vi "LINC Command Lookup.vi"(8 "error in (no error)":errorcluster, 11 "LINC session":refnum<class "LINC.lvclass">) -> (0 "error out":errorcluster, 1 "cmd data":string, 2 "cmd name":string, 3 "dup LINC session":refnum<class "LINC.lvclass">, 4 "cmd origin":T1, 5 "cmd header fields":i32, 6 "cmd GUID":string)   [LabVIEW 2018, in "STEPkgDriver_LINC.lvlib" / "LINC.lvclass"]
uses:
  LINC.lvclass
  STEPkgDriver_LINC.lvlib
  LINC Global Mode.ctl
  LINC Global Config Mode.ctl
  LINC Command Origin.ctl
  LINC Command.ctl
  LINC Global Handshake Mode.ctl
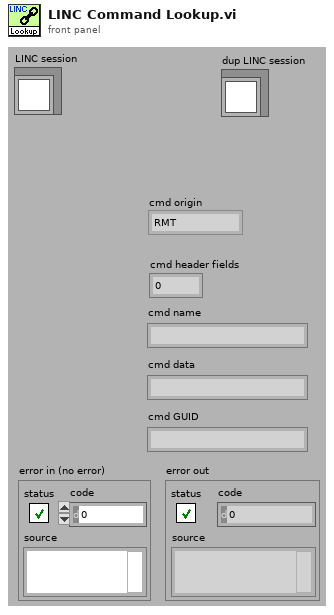
[diagram p1: front panel]
types:
  T1 = typedef "STEPkgDriver_LINC.lvlib/LINC Command Origin.ctl" = enum8{"RMT", "LCL"}
  T2 = typedef "STEPkgDriver_LINC.lvlib/LINC Global Handshake Mode.ctl" = enum16{"INIT", "CLEAR", "ADD_COMMAND", "RMV_COMMAND", "CLR_HANDSHAKE", "SET_HANDSHAKE", "GET_HANDSHAKE"}
  T3 = typedef "STEPkgDriver_LINC.lvlib/LINC Command.ctl" = cluster{"command origin":T1, "command":string, "command data":string}
  T4 = typedef "STEPkgDriver_LINC.lvlib/LINC Global Config Mode.ctl" = enum16{"INIT", "CLEAR", "SET_CMD_CB", "SET_TLM_CB", "SET_CMD_FIELDS", "SET_TLM_FIELDS", "SET_ID", "GET_CONFIG"}
  T5 = typedef "STEPkgDriver_LINC.lvlib/LINC Global Mode.ctl" = enum16{"INIT", "CLEAR", "ADD_PKT_HDR", "ADD_PKT", "GET_PKT_NAMES", "GET_PKT_DESC", "GET_PKT_HDR", "GET_PKT", "SET_PKT", "SET_DATA", "SIM_EN", "SIM_DS"}
  T6 = typedef "STEPkgDriver_LINC.lvlib/LINC Config.ctl" = cluster{"cmd callback":refnum<vi>, "tlm callback":refnum<vi>, "cmd ID bitoffset":i32, "cmd ID bitsize":i32, "cmd IDs":i32[], "tlm ID bitoffset":i32, "tlm ID bitsize":i32, "tlm IDs":i32[], "cmd header fields":i32, "tlm header fields":i32, "tlm header size":i32}
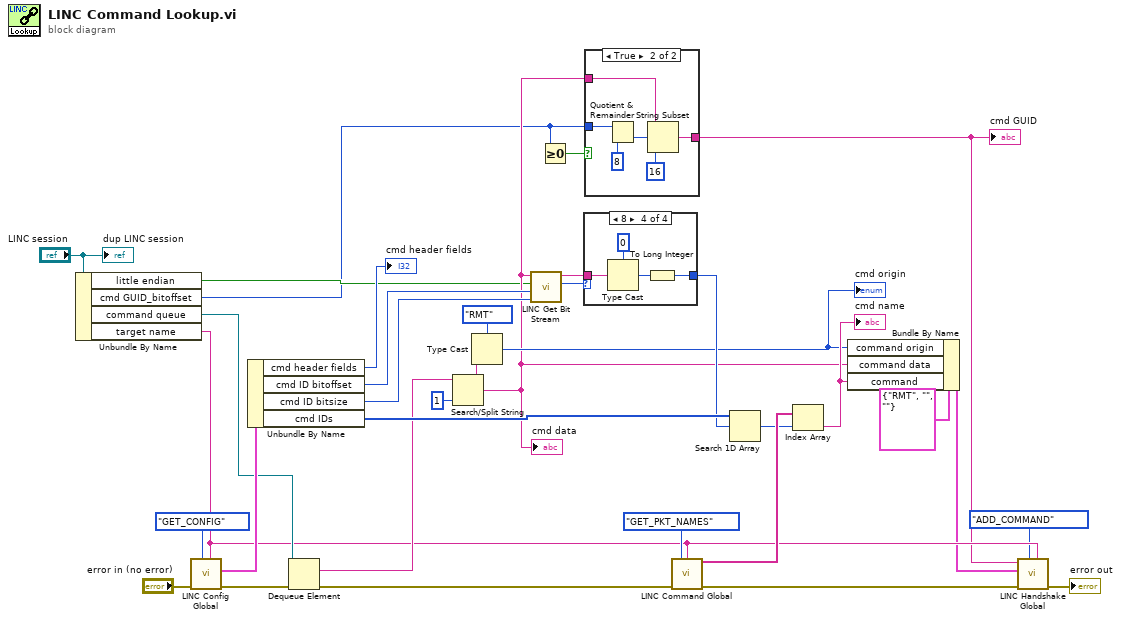
[diagram p0: block diagram]
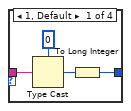
[diagram p3: hidden frame]
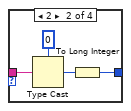
[diagram p4: hidden frame]
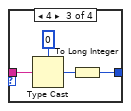
[diagram p5: hidden frame]
diagram:
  n1 = Unbundle By Name("LINC session") -> ("little endian"=w6:bool, "cmd GUID_bitoffset"=w5:i32, "command queue"=w20:refnum<queue>, "target name"=w19:string)
  n2 = call "LINC Config Global.vi"("target name"=w19, "mode"=LINC_Global_Config_Mode."GET_CONFIG", "error in (no error)"="error in (no error)") -> ("error out"=w27:errorcluster, "config out"=w28:T6)  [unwired: 7 in]
  n3 = Unbundle By Name(w28) -> ("cmd header fields"=→"cmd header fields":i32, "cmd ID bitoffset"=w15:i32, "cmd ID bitsize"=w14:i32, "cmd IDs"=w32:i32[])
  n4 = Dequeue Element(queue=w20, error in (no error)=w27) -> (element=w26:string, error out=w23:errorcluster)  [unwired: 1 in, 2 out]
  n5 = Search/Split String(string=w26, offset (0)=1) -> (substring before match=w24:string, match + rest of string=w7:string)  [unwired: 1 in, 1 out]
  "cmd data" <- w7
  n6 = Type Cast(type=LINC_Command_Origin."RMT" ("cmd origin"), x=w24) -> (*(type *) &x=w9:T1)
  "cmd origin" <- w9
  n7 = call "LINC Get Bit Stream.vi"("bit size"=w14, "bit offset"=w15, "little endian"=w6, "data in"=w7) -> ("bytes"=w13:i32, "data out"=w12:string)  [unwired: 6 in]
  n8 = Greater Or Equal To 0?(x=w5) -> (x >= 0?=w4:bool)
  n9 = case shown="8" w13 {
    tunnel: w12 -> [w38 w42 w46 w50]
    tunnel: [w35 w39 w43 w47] -> w11
    frame 1, Default {
      n10 = Type Cast(type=u8 0, x=w38) -> (*(type *) &x=w36:u8)
      n11 = To Long Integer(number=w36) -> (32bit integer=w35:i32)
    }
    frame 2 {
      n12 = Type Cast(type=u16 0, x=w42) -> (*(type *) &x=w40:u16)
      n13 = To Long Integer(number=w40) -> (32bit integer=w39:i32)
    }
    frame 4 {
      n14 = Type Cast(type=u32 0, x=w46) -> (*(type *) &x=w44:u32)
      n15 = To Long Integer(number=w44) -> (32bit integer=w43:i32)
    }
    frame 8 {
      n16 = Type Cast(type=u64 0, x=w50) -> (*(type *) &x=w48:u64)
      n17 = To Long Integer(number=w48) -> (32bit integer=w47:i32)
    }
  }
  n18 = case shown="True" w4 {
    tunnel: w7 -> [_ w56]
    tunnel: w5 -> [_ w55]
    tunnel: [_ w51] -> w1
    frame False {
    }
    frame True {
      n19 = Quotient & Remainder(x=w55, y=8) -> (floor(x/y)=w53:i32)  [unwired: 1 out]
      n20 = String Subset(string=w56, offset (0)=w53, length (rest)=16 ("length (rest)")) -> (substring=w51:string)
    }
  }
  "cmd GUID" <- w1
  n21 = call "LINC Command Global.vi"("mode"=LINC_Global_Mode."GET_PKT_NAMES", "target name"=w19, "error in (no error)"=w23) -> ("values out"=w34:string[], "error out"=w22:errorcluster)  [unwired: 8 in, 3 out]
  n22 = Search 1D Array(1D array=w32, element=w11) -> (index of element=w31:i32)  [unwired: 1 in]
  n23 = Index Array(array=w34, index=w31) -> (element=w18:string)
  "cmd name" <- w18
  n24 = Bundle By Name(cluster=T3 {"command origin"=enum."RMT", "command"="", "command data"=""} ("housekeeping in"), "command origin"=w9, "command data"=w7, "command"=w18) -> (w3:T3)
  n25 = call "LINC Handshake Global.vi"("target name"=w19, "mode"=LINC_Global_Handshake_Mode."ADD_COMMAND", "error in (no error)"=w22, "command in"=w3, "GUID"=w1) -> ("error out"=→"error out":errorcluster)  [unwired: 3 in, 3 out]
  "dup LINC session" <- "LINC session"
